vi "NIRFSG_Close.vi"(8 "error in (no error)":errorcluster, 11 "instrument handle":refnum<k15>) -> (0 "error out":errorcluster)   [LabVIEW 2015]
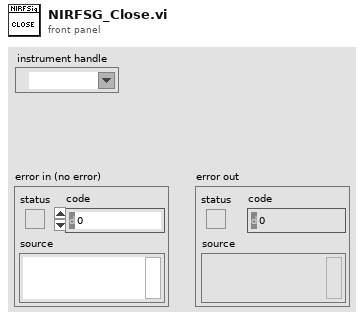
[diagram p1: front panel]
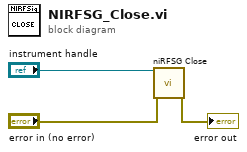
[diagram p0: block diagram]
diagram:
  n1 = call <instrlib>:"niRFSG Close.vi"("instrument handle"="instrument handle", "error in"="error in (no error)") -> ("error out"=→"error out":errorcluster)  [unwired: 13 in]
